vi "Test_WriteValue_InvalidType_Error.vi"(8 "error in (no error)":errorcluster, 11 "TestCase in":refnum<class "TestRingStringsBinding.lvclass">) -> (0 "error out":errorcluster, 3 "TestCase out":refnum<class "TestRingStringsBinding.lvclass">)   [LabVIEW 2017, in "TestRingStringsBinding.lvclass"]
uses:
  TestRingStringsBinding.lvclass
  Source/Concrete/RingStringsBinding/RingStringsBinding.lvclass
  C:/Git/composed-transport/Source/ITransport/ITransport.lvclass
  Source/ITransport/ITransport.lvclass
panel:
  out "Return Error":errorcluster
  in  "Ring":u16(ring)
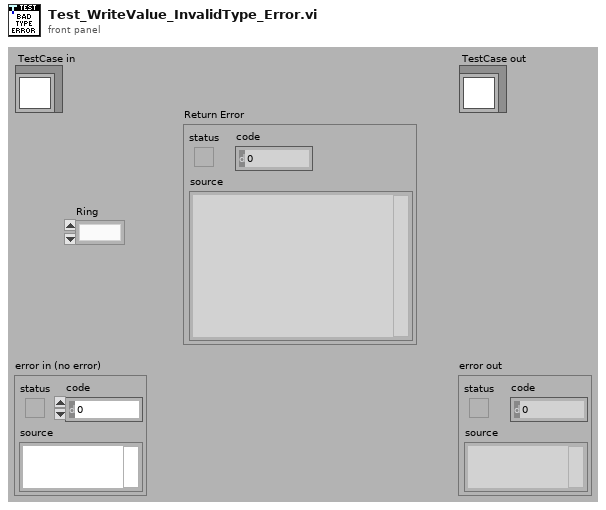
[diagram p1: front panel]
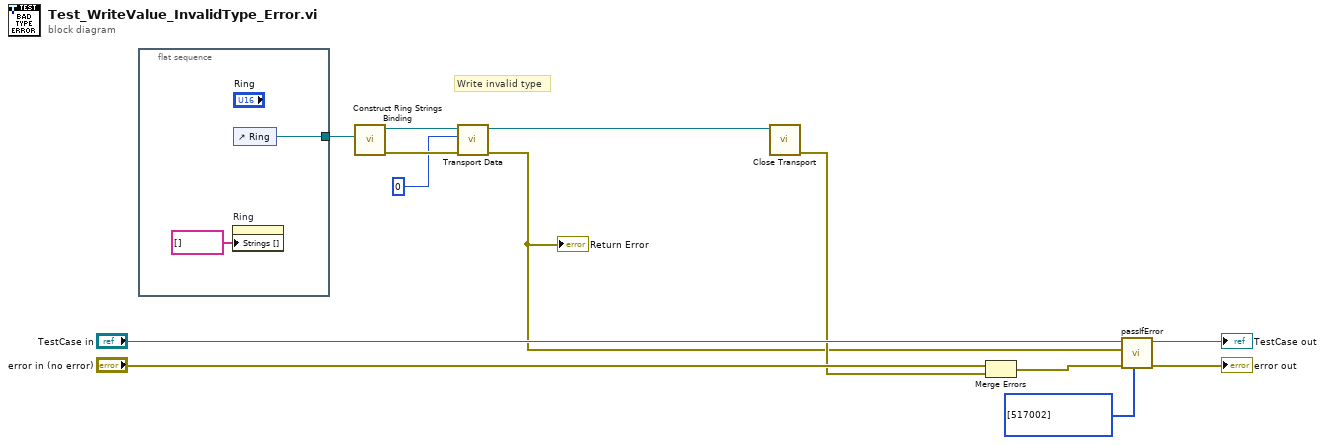
[diagram p0: block diagram]
diagram:
  # "Write invalid type"
  n1 = flat-sequence {
    tunnel: [w15] -> w5
    frame #0 {
      n2 = property on="Ring" class="Ring (strict)"("Strings []"=string[] []) -> ()  [unwired: 2 in, 2 out]
      n3 = control-ref of="Ring"() -> (w15:refnum<vi>)
    }
  }
  n4 = call "Construct Ring Strings Binding.vi"("Ring Refnum"=w5) -> ("error out"=w7:errorcluster, "RingStringsBinding"=w9:refnum<class "RingStringsBinding.lvclass">)  [unwired: 9 in]
  n5 = call "Transport Data.vi"("error in (no error)"=w7, "Value"=0, "ITransport in"=w9) -> ("error out"=w2:errorcluster, "ITransport out"=w6:refnum<class "RingStringsBinding.lvclass">)  [unwired: 7 in]
  "Return Error" <- w2
  n6 = call-dynamic "Close Transport.vi"("ITransport in"=w6) -> ("error out"=w4:errorcluster)  [unwired: 10 in]
  n7 = Merge Errors("error in (no error)", w4) -> (w8:errorcluster)
  n8 = call-dynamic "passIfError.vi"("passing error codes (default = any error code)"=i32[] [517002], "error in (no error)"=w8, "error"=w2, "TestCase in"="TestCase in") -> ("error out"=→"error out":errorcluster, "TestCase out"=→"TestCase out":refnum<class "TestRingStringsBinding.lvclass">)  [unwired: 6 in]
